vi "SrsQcm200FandR_MODIFIED 2017-11-12.vi"(0 "VISA in":refnum<visa-resource-name>="GPIB0::3::INSTR", 11 "error in (no error)":errorcluster) -> (4 "VISA out":refnum<visa-resource-name>, 6 "Frequency out":dbl format="%.6f", 10 "Resistance out":dbl format="%.6f", 15 "error out":errorcluster)   [LabVIEW 2014]
doc: "This VI returns the QCM200 frequency and resistance values together.\n\nCopyright 2004 Stanford Research Systems"
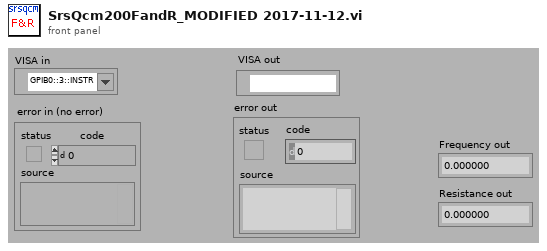
[diagram p1: front panel]
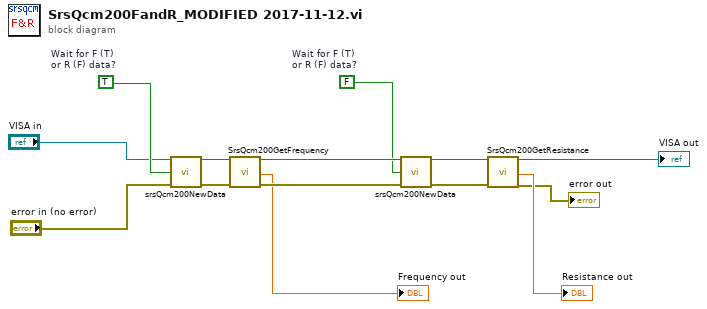
[diagram p0: block diagram]
diagram:
  w11 = FALSE  # Wait for F (T) or R (F) data?
  w10 = TRUE  # Wait for F (T) or R (F) data?
  n1 = call "srsQcm200NewData.vi"("VISA in"="VISA in", "Wait for F (T)\nor R (F) data?"=w10, "error in (no error)"="error in (no error)") -> ("VISA out"=w14:refnum<visa-resource-name>, "error out"=w4:errorcluster)  [unwired: 11 in]
  n2 = call "SrsQcm200GetFrequency.vi"("VISA in"=w14, "error in (no error)"=w4) -> ("VISA out"=w12:refnum<visa-resource-name>, "Frequency out"=→"Frequency out":dbl, "error out"=w13:errorcluster)  [unwired: 15 in]
  n3 = call "srsQcm200NewData.vi"("VISA in"=w12, "Wait for F (T)\nor R (F) data?"=w11, "error in (no error)"=w13) -> ("VISA out"=w7:refnum<visa-resource-name>, "error out"=w3:errorcluster)  [unwired: 11 in]
  n4 = call "SrsQcm200GetResistance.vi"("VISA in"=w7, "error in (no error)"=w3) -> ("VISA out"=→"VISA out":refnum<visa-resource-name>, "Resistance out"=→"Resistance out":dbl, "error out"=→"error out":errorcluster)  [unwired: 15 in]
